vi "CallUserScripting.vi"(8 "error in":errorcluster, 11 "MultiDimArrElemScripter in":refnum<class "MultiDimArrElemScripter.lvclass">) -> (0 "error out":errorcluster, 3 "MultiDimArrElemScripter out":refnum<class "MultiDimArrElemScripter.lvclass">)   [LabVIEW 2021, in "MemberVICreation.lvlib" / "MultiDimArrElemScripter.lvclass"]
doc: "This VI provides an opportunity for users to add scripting code of their own to modify the scripting process even if they do not have the password to the VIs in the scripting. Each overriding class should call out to an empty subVI, one that is not a member of the class, that users can edit to put in their own scripting behavior."
uses:
  <resource>/Framework/Providers/LVClassLibrary/NewAccessors/MultiDimArrElemScripter/MultiDimArrElemScripter.lvclass
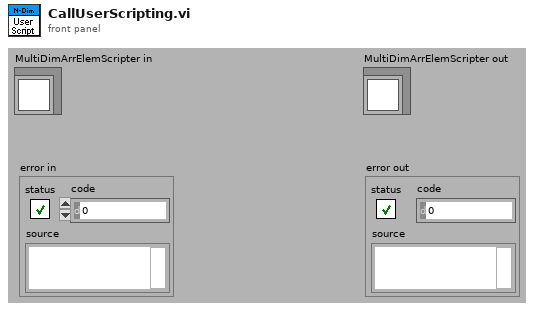
[diagram p1: front panel]
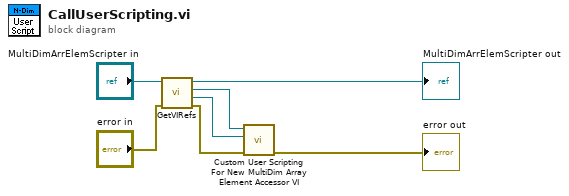
[diagram p0: block diagram]
diagram:
  n1 = call-dynamic "GetVIRefs.vi"("error in (no error)"="error in", "BaseAccessorScripter in"="MultiDimArrElemScripter in") -> ("error out"=w3:errorcluster, "Write VI"=w2:refnum<vi>, "Read VI"=w4:refnum<vi>, "BaseAccessorScripter out"=→"MultiDimArrElemScripter out":refnum<class "MultiDimArrElemScripter.lvclass">)  [unwired: 6 in]
  n2 = call <resource>:"Custom User Scripting For New MultiDim Array Element Accessor VI.vi"("error in"=w3, "Write VI"=w2, "Read VI"=w4) -> ("error out"=→"error out":errorcluster)  [unwired: 8 in]
